vi "SetStepAmplitudeNegative.vi"(0 "CmdLib In":refnum<k24>, 5 "Output Refnum In":refnum<vi>, 7 "Axis":i32, 9 "Step Amplitude":i32, 11 "error in (no error)":errorcluster) -> (4 "CmdLib Out":refnum<k24>, 6 "SetStepAmplitudeNegative":bool, 15 "error out":errorcluster)   [LabVIEW 2013]
uses:
  C:/Code/Apps/Utilities/AG-UC2-UC8/AG-UC2-UC8/Install/Samples/LabVIEW/LabVIEW 2013/CmdLibAgilis.dll
  CmdLibAgilis.dll
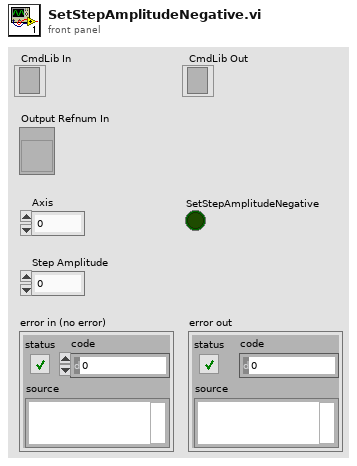
[diagram p1: front panel]
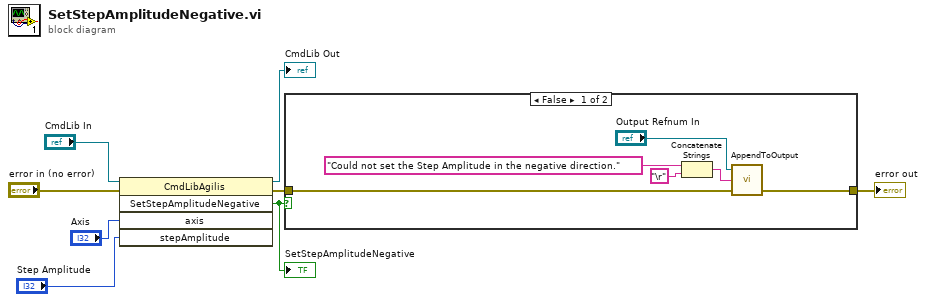
[diagram p0: block diagram]
diagram:
  n1 = invoke class="CmdLibAgilis" method="SetStepAmplitudeNegative"(reference="CmdLib In", error in="error in (no error)", "axis"="Axis", "stepAmplitude"="Step Amplitude") -> (reference out=→"CmdLib Out":refnum<k24>, error out=w2:errorcluster, "SetStepAmplitudeNegative"=w3:bool)  [unwired: 1 in, 2 out]
  "SetStepAmplitudeNegative" <- w3
  n2 = case shown="False" w3 {
    tunnel: w2 -> [w12 w15]
    tunnel: [w11 w15] -> w1
    frame False {
      n3 = Concatenate Strings("Could not set the Step Amplitude in the negative direction.", "\r") -> (w10:string)
      n4 = call "AppendToOutput.vi"("error in"=w12, "Input String"=w10, "Output Refnum In"="Output Refnum In") -> ("error out"=w11:errorcluster)  [unwired: 1 in, 1 out]
    }
    frame True {
    }
  }
  "error out" <- w1
